vi "LV SCISDK Get Parameter U Integer.vi"(8 "error in (no error)":errorcluster, 10 "handle":u64, 11 "Path":string) -> (0 "error out":errorcluster, 1 "function return":i32, 2 "handle out":u64, 3 "value":u32)   [LabVIEW 2021]
doc: "SCISDKLABVIEW_DLL_API int LV_SCISDK_GetParameterUInteger(char* Path, unsigned int* value, void* handle);"
uses:
  SciSDK_Labview.dll
  SciSDK_Labview.lvlib
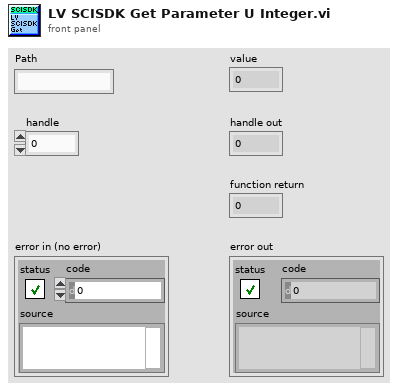
[diagram p1: front panel]
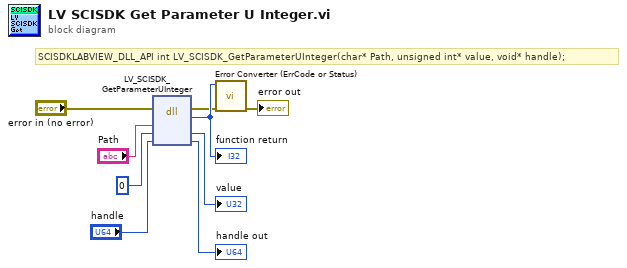
[diagram p0: block diagram]
diagram:
  # "SCISDKLABVIEW_DLL_API int LV_SCISDK_GetParameterUInteger(char* Path, unsigned int* value, void* handle);"
  n1 = dll-call lib="C:/git/scisdk/wrapper/LabView/SciSDK_Labview.*" fn="LV_SCISDK_GetParameterUInteger"(error in="error in (no error)", "Path"="Path", "value"=u32 0, "handle"="handle") -> (error out=w2:errorcluster, w9:i32, "value"=→"value":u32, "handle"=→"handle out":u64)  [unwired: 3 in, 1 out]
  "function return" <- w9
  n2 = call "Error Converter (ErrCode or Status).vi"("error in (no error)"=w2, "error code"=w9) -> ("error out"=→"error out":errorcluster)  [unwired: 9 in]
